vi "CSTK_BuildApplication_Manager_BuildAction_Core.vi"(10 "错误输入（无错误）":errorcluster, 11 "项目路径":path) -> (2 "错误输出":errorcluster, 3 "SavePath":path)   [LabVIEW 2015, in "CSTK_BuildApplication_Manager.lvlib"]
uses:
  CSTK_BuildApplication_Manager.lvlib
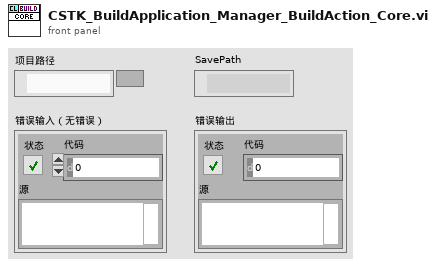
[diagram p1: front panel]
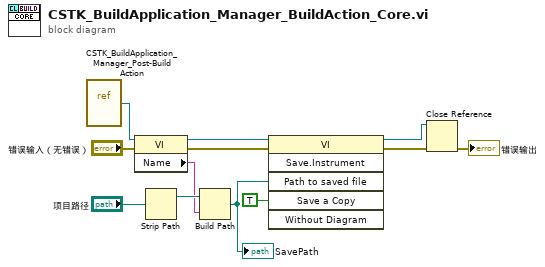
[diagram p0: block diagram]
diagram:
  n1 = vi-ref "CSTK_BuildApplication_Manager_Post-Build Action.vi"() -> (w11:refnum<vi>)
  n2 = property class="VI"(reference=w11, error in="错误输入（无错误）") -> (reference out=w3:refnum<vi>, error out=w2:errorcluster, "Name"=w1:string)
  n3 = Strip Path(path="项目路径") -> (stripped path=w8:path)  [unwired: 1 out]
  n4 = Build Path(base path=w8, name or relative path=w1) -> (appended path=w7:path)
  "SavePath" <- w7
  n5 = invoke class="VI" method="Save.Instrument"(reference=w3, error in=w2, "Path to saved file"=w7, "Save a Copy"=TRUE ("保存副本")) -> (reference out=w5:refnum<vi>, error out=w6:errorcluster)  [unwired: 2 in, 4 out]
  n6 = Close Reference(reference=w5, error in (no error)=w6) -> (error out=→"错误输出":errorcluster)
